vi "pratik2-case2.vi"() -> ()   [LabVIEW 2024]
panel:
  out "x*y":dbl
  out "x+y":u32
  out "Byte 4":bool[](array[boolean])
  out "number":u32
  in  "Input String":string
  out "RESOLUTION (AMPER)":dbl format="%#_5g"
  out "RESOLUTION (mA)":dbl
  out "Byte2-subarray":bool[](array[boolean])
  out "CONFIGURATION VERSION":string
  out "Configuration Device ID":u32
  out "Configuration Version LSB":u32
  out "Configuration Version MSB":u32
  out "number in decimal":u32
  out "Byte 3":bool[](array[boolean])
  out "Byte 2":bool[](array[boolean])
  out "LSB(8-16)":bool[](array[boolean])
  out "MSB(0-7)":bool[](array[boolean])
  out "Array":bool[](array[boolean])
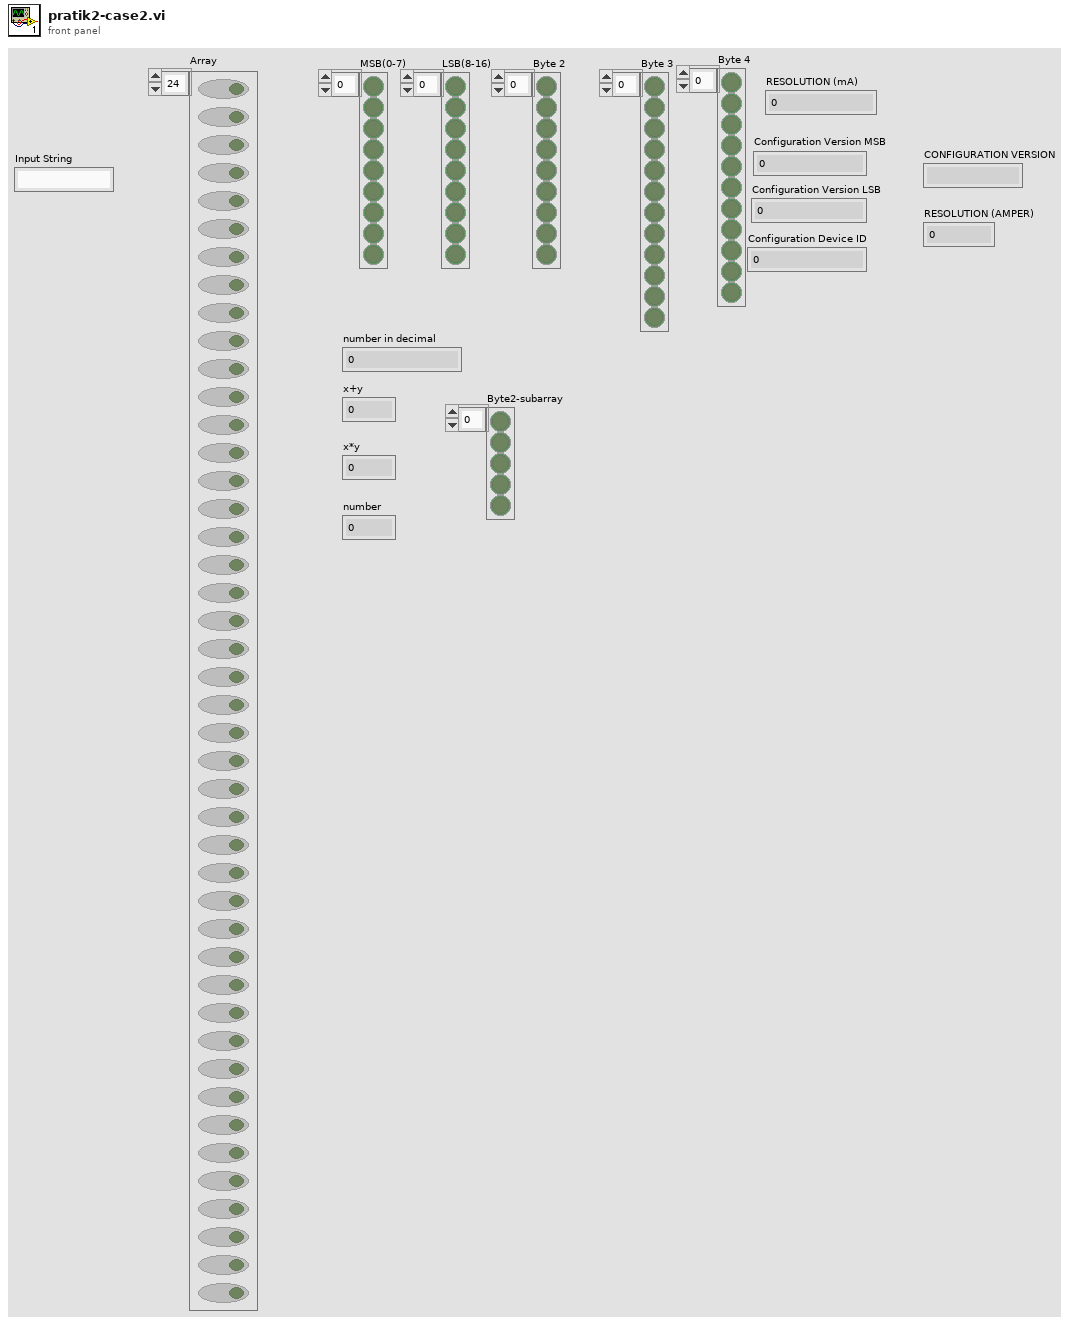
[diagram p1: front panel]
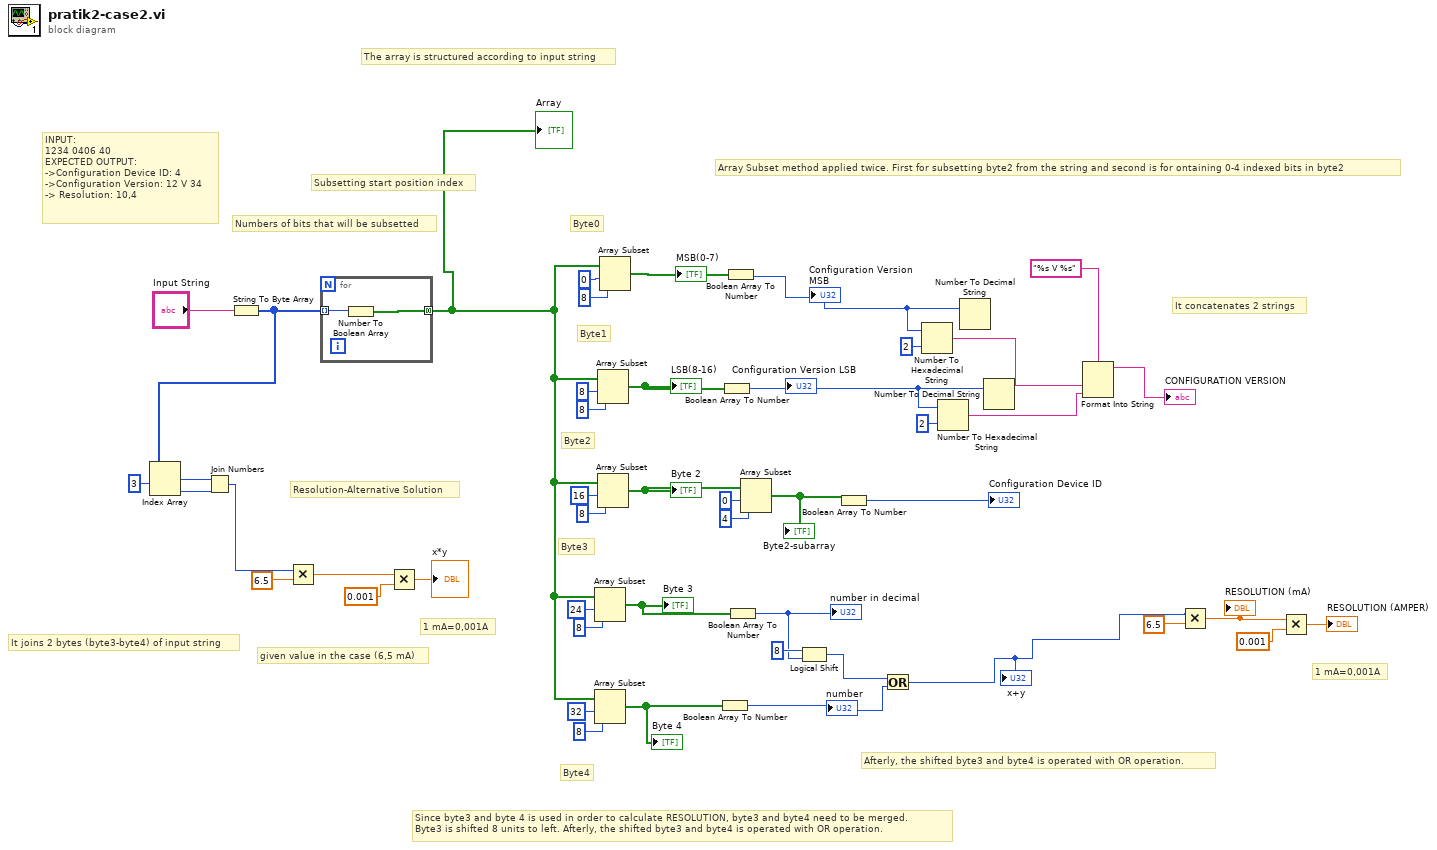
[diagram p0: block diagram]
diagram:
  # "Numbers of bits that will be subsetted"
  # "Subsetting start position index"
  # "Afterly, the shifted byte3 and byte4 is operated with OR operation."
  # "Since byte3 and byte 4 is used in order to calculate RESOLUTION, byte3 and byte4 need to be merged. \nByte3 is shifted 8 units to left. Afterly, the shifted byte3 and byte4 is operated with OR operation."
  # "Array Subset method applied twice. First for subsetting byte2 from the string and second is for ontaining 0-4 indexed bits in byte2"
  # "It concatenates 2 strings"
  # "given value in the case (6,5 mA)"
  # "It joins 2 bytes (byte3-byte4) of input string"
  # "Resolution-Alternative Solution"
  # "Byte4"
  # "Byte3"
  # "Byte2"
  # "Byte1"
  # "Byte0"
  # "The array is structured according to input string"
  # "INPUT:\n1234 0406 40\nEXPECTED OUTPUT:\n->Configuration Device ID: 4\n->Configuration Version: 12 V 34\n-> Resolution: 10,4"
  # "1 mA=0,001A"
  # "1 mA=0,001A"
  n1 = String To Byte Array(string="Input String") -> (unsigned byte array=w9:u8[])
  n2 = Index Array "Index Array"(array=w9, index #1=3 ("index")) -> (element #1=w7:u8, element #2=w6:u8)  [unwired: 1 in]
  n3 = Join Numbers(hi=w7, lo=w6) -> ((hi.lo)=w2:u16)
  n4 = Multiply(x=w2, y=6.5) -> (x*y=w4:dbl)
  n5 = for {
    tunnel: w9 -> [w49] mode=indexing
    tunnel: [w48] -> w17 mode=concatenating
    n6 = Number To Boolean Array(number=w49) -> (Boolean array=w48:bool[])
  }
  "Array" <- w17
  n7 = Multiply(x=w4, y=0.001) -> (x*y=→"x*y":dbl)
  n8 = Array Subset "Array Subset"(array=w17, index=24, length=8) -> (w16:bool[])
  "Byte 3" <- w16
  n9 = Array Subset "Array Subset"(array=w17, index=32, length=8) -> (w15:bool[])
  "Byte 4" <- w15
  n10 = Array Subset "Array Subset"(array=w17, index=8, length=8) -> (w39:bool[])
  "LSB(8-16)" <- w39
  n11 = Array Subset "Array Subset"(array=w17, index=16, length=8) -> (w34:bool[])
  "Byte 2" <- w34
  n12 = Array Subset "Array Subset"(array=w17, index=0, length=8) -> (w40:bool[])
  "MSB(0-7)" <- w40
  n13 = Boolean Array To Number(Boolean array=w15) -> (number=w11:u32)
  "number" <- w11
  n14 = Boolean Array To Number(Boolean array=w39) -> (number=w20:u32)
  "Configuration Version LSB" <- w20
  n15 = Boolean Array To Number(Boolean array=w40) -> (number=w25:u32)
  "Configuration Version MSB" <- w25
  n16 = Boolean Array To Number(Boolean array=w16) -> (number=w13:u32)
  "number in decimal" <- w13
  n17 = Array Subset(array=w34, index=0, length=4) -> (w31:bool[])
  "Byte2-subarray" <- w31
  n18 = Logical Shift(y=i16 8, x=w13) -> (x << y=w12:u32)
  n19 = Boolean Array To Number(Boolean array=w31) -> (number=→"Configuration Device ID":u32)
  n20 = Or(x=w12, y=w11) -> (x .or. y?=w10:u32)
  "x+y" <- w10
  n21 = Number To Hexadecimal String(1:i16 2 ("width (-)"), 2:w25) -> (0:w24:string)
  n22 = Number To Hexadecimal String(1:i16 2 ("width (-)"), 2:w20) -> (0:w21:string)
  n23 = Number To Decimal String(number=w25) -> ()  [unwired: 1 in, 1 out]
  n24 = Number To Decimal String(number=w20) -> ()  [unwired: 1 in, 1 out]
  n25 = Format Into String "Format Into String"(format string="%s V %s", w24, w21) -> (resulting string=→"CONFIGURATION VERSION":string)  [unwired: 2 in, 1 out]
  n26 = Multiply(x=w10, y=6.5) -> (x*y=w29:dbl)
  "RESOLUTION (mA)" <- w29
  n27 = Multiply(x=w29, y=0.001) -> (x*y=→"RESOLUTION (AMPER)":dbl)
